vi "Obtain Message Queue.vi"(7 "max queue size (-1, unlimited)":i32=-1, 8 "error in (no error)":errorcluster) -> (0 "error out":errorcluster, 3 "Message Queue":refnum<queue>)   [LabVIEW 2018, in "Message Queue.lvlib"]
doc: "Create a queue with the Message Cluster data type."
uses:
  Message Queue.lvlib
  Message Cluster.ctl
  Message.ctl
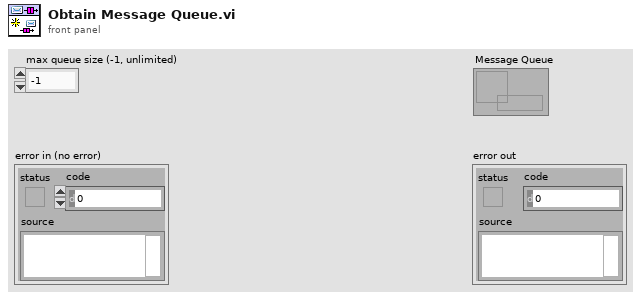
[diagram p1: front panel]
types:
  T1 = typedef "Message Queue.lvlib/Message Cluster.ctl" = cluster{"Message":T2, "Message Data":variant}
  T2 = typedef "Message Queue.lvlib/Message.ctl" = enum16{"Initialize", "Initialize UI Refs", "Disable Controls", "Enable UI Controls", "Connect RT", "Get Control Mode from RT", "Send Control Mode to UI", "Update Control Mode", "Get Config from RT", "Send Config to UI", "Update Parameters", "Change Parameters", "Calibrate Config", "Update Calibration", "Change Valve State", "Get Valve Status from RT", "Send Valve Status to UI", "Update Valve Status", "Inital UI Values", "Disconnect RT", "Close Connection", "Disconnect UI", "Run Mode", "Stop ALL", "Change Control Mode", "Skid Manual", "Computer Manual", "Step Automated", "Fully Automated", "Reset", "Pumps Command", "Pump State Changed", "Critical Error", "Log-Only Error", "Non-Critical Error", "RT Error", "Update System Status", "Update DI Status", "Clear System Status", "Update Warning", "Clear Warning", "Upate Timeout", "Update Reset Status", "Waiting", "Verify Password", "Manual Cleaning Process", "Update Manual Cleaning Process", "Cal - Body", "Cal - US", "Cal - Update Parameters", "Propotional Update", "Exit", "---Copy This Frame---"}
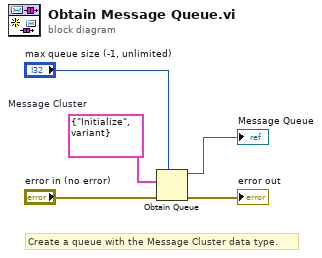
[diagram p0: block diagram]
diagram:
  w5 = T1 {"Message"=enum."Initialize", "Message Data"=variant}  # Message Cluster
  # "Create a queue with the Message Cluster data type."
  n1 = Obtain Queue(max queue size (-1, unlimited)="max queue size (-1, unlimited)", element data type=w5, error in (no error)="error in (no error)") -> (queue out=→"Message Queue":refnum<queue>, error out=→"error out":errorcluster)  [unwired: 2 in, 1 out]
